vi "Connect.vi"(9 "Xwave Connection":T2={"addr"="192.168.2.51", "Main Port"=3000, "UDP Port"=3001}) -> (0 "error Out":errorcluster, 2 "Conn":T1, 3 "Connected?":bool)   [LabVIEW 2014]
uses:
  type_def/Conns_Params.ctl
  ConsCluster.ctl
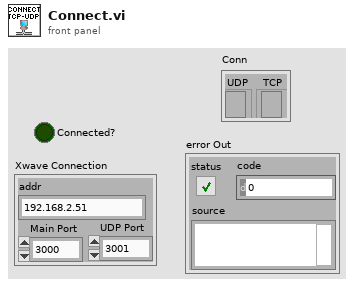
[diagram p1: front panel]
types:
  T1 = typedef "ConsCluster.ctl" = cluster{"UDP":refnum<k16>, "TCP":refnum<k5>}
  T2 = typedef "Conns_Params.ctl" = cluster{"addr":string, "Main Port":u16, "UDP Port":u16}
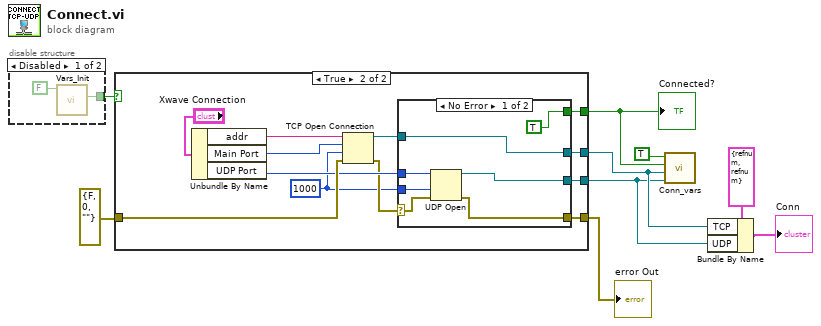
[diagram p0: block diagram]
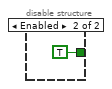
[diagram p2: hidden frame]
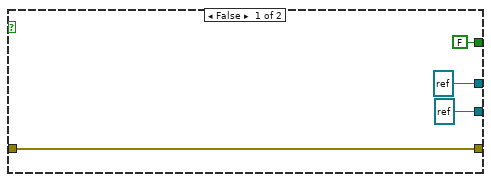
[diagram p3: hidden frame]
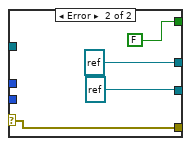
[diagram p4: hidden frame]
diagram:
  n1 = disable-structure shown="Disabled" {
    disable-tunnel: [w11 TRUE ("Init? Out")] -> w7
    frame Disabled {
      n2 = call "Vars_Init.vi"("WriteVars?"=FALSE) -> ("Init? Out"=w11:bool)  [unwired: 9 in, 1 out]
    }
    frame Enabled {
    }
  }
  n3 = case shown="True" w7 {
    tunnel: errorcluster {"status"=FALSE, "code"=0, "source"=""} ("error out") -> [w16 w27]
    tunnel: [w16 w28] -> w9
    tunnel: [FALSE ("WriteVars?") w19] -> w5
    tunnel: [refnum<k16> refnum ("UDPConn in") w18] -> w2
    tunnel: [refnum<k5> refnum ("TCP Conn In") w17] -> w3
    frame False {
    }
    frame True {
      w20 = 1000 ("timeout ms (25000)")
      n4 = Unbundle By Name("Xwave Connection") -> ("addr"=w25:string, "Main Port"=w24:u16, "UDP Port"=w22:u16)
      n5 = TCP Open Connection(address=w25, remote port or service name=w24, timeout ms (60000)=w20, error in (no error)=w27) -> (connection ID=w23:refnum<k5>, error out=w21:errorcluster)  [unwired: 1 in]
      n6 = case shown="No Error" w21 {
        selector: w21 -> [w34 w39]
        tunnel: [w32 w39] -> w28
        tunnel: w23 -> [w30 _]
        tunnel: w22 -> [w35 _]
        tunnel: w20 -> [w33 _]
        tunnel: [TRUE ("WriteVars?") FALSE ("WriteVars?")] -> w19
        tunnel: [w29 refnum<k16> refnum ("UDPConn in")] -> w18
        tunnel: [w30 refnum<k5> refnum ("TCP Conn In")] -> w17
        frame No Error {
          n7 = UDP Open(8:w34, 9:w33, 11:w35) -> (port=w29:refnum<k16>, 0:w32:errorcluster)  [unwired: 2 in, 1 out]
        }
        frame Error {
        }
      }
    }
  }
  "error Out" <- w9
  "Connected?" <- w5
  n8 = call "Conn_vars.vi"("UDPConn In"=w2, "TCP Conn In"=w3, "Connected_In"=w5, "WriteVars?"=TRUE) -> ()  [unwired: 5 in, 3 out]
  n9 = Bundle By Name(cluster=T1 {"UDP"=refnum, "TCP"=refnum} ("Conn"), "TCP"=w3, "UDP"=w2) -> (→"Conn":T1)
